vi "Write Measurement.vi"(8 "error in (no error)":errorcluster, 10 "Measurement":string, 11 "DataPoint in":refnum<class "DataPoint.lvclass">) -> (0 "error out":errorcluster, 3 "DataPoint out":refnum<class "DataPoint.lvclass">)   [LabVIEW 2018, in "InfluxDB Client.lvlib" / "DataPoint.lvclass"]
uses:
  DataPoint.lvclass
  DataPoint.lvclass/DataPoint.ctl
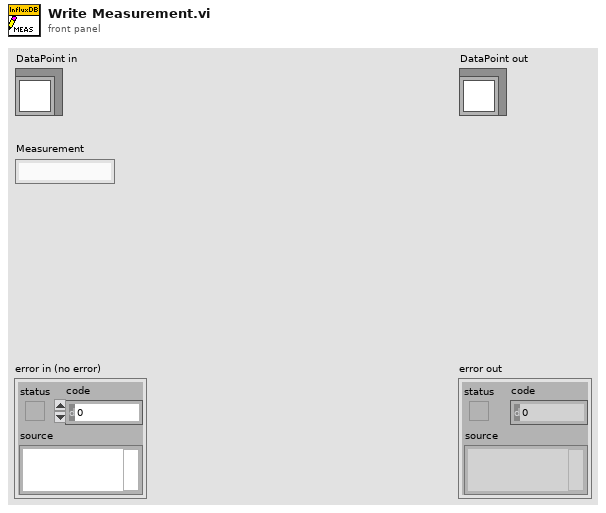
[diagram p1: front panel]
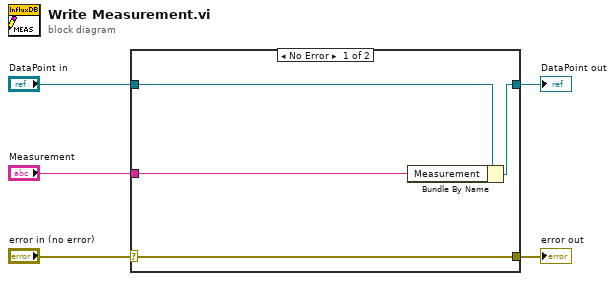
[diagram p0: block diagram]
diagram:
  n1 = case shown="No Error" "error in (no error)" {
    selector: "error in (no error)" -> [w9 w10]
    tunnel: [w9 w10] -> w4
    tunnel: [w7 w11] -> w2
    tunnel: "DataPoint in" -> [w8 w11]
    tunnel: "Measurement" -> [w6 _]
    frame No Error {
      n2 = Bundle By Name(cluster=w8, "Measurement"=w6) -> (w7:refnum<class "DataPoint.lvclass">)
    }
    frame Error {
    }
  }
  "error out" <- w4
  "DataPoint out" <- w2
